vi "GenFPGActrlRef.vi"(4 "DSA excitation":dbl, 6 "Ref Ch.":T2, 7 "Current Time [s]":dbl, 8 "error in (no error)":errorcluster, 9 "Z,ThX,ThY Ref_Cluster":T3 {"Twist_ref [V]" step=0.1; "Bend_ref [V]" step=0.1}, 10 "Reference Offset":T4={"phase"=0.0, "amplitude"=1.0, "frequency"=1.0, "offset"=1.0, "Signal"=enum."Sine"} {"offset" format="%0.2f"; "frequency" format="%0.2f"; "amplitude" format="%0.2f"; "phase" format="%0.2f"}, 11 "FPGA Interface":T1) -> (0 "error out":errorcluster, 2 "Ref Signal":dbl[](array[numeric]), 3 "FPGA VI Reference Out":T1)   [LabVIEW 2017]
doc: "Generate reference signal for the FPGA controller and send params to FPGA"
uses:
  Components/SignalGen/SignalGen.lvlib
  <vilib>/rvi/interface/nirviReadWriteControl/nirviReadWriteControl.xnode
  TypeDefs/FPGA VI Reference.ctl
  FPGA Bitfiles/flexlab_FPGATarget_Tbeamrawv2MainVI_U8ISWGKWIPM.lvbitx
  NiFpgaLv.dll
  <vilib>/Utility/error.llb/Error Cluster From Error Code.vi
  <vilib>/rvi/errors/niLvFpgaAdjustHostInterfaceError.vi
  Components/SignalGen/SignalGenParams_Cluster.ctl
  TypeDefs/BendTwist_Ref_Cluster.ctl
  TypeDefs/RefChEnum.ctl
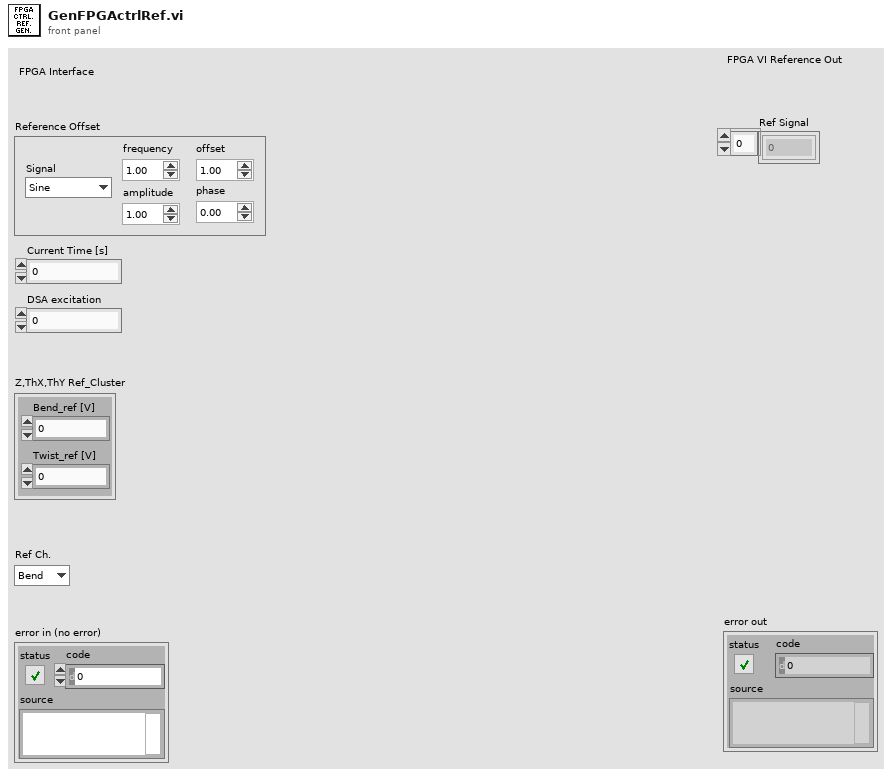
[diagram p1: front panel]
types:
  T1 = typedef "FPGA VI Reference.ctl" = refnum<k20>
  T2 = typedef "RefChEnum.ctl" = enum16{"Bend", "Twist"}
  T3 = typedef "BendTwist_Ref_Cluster.ctl" = cluster{"Bend_ref [V]":dbl, "Twist_ref [V]":dbl}
  T4 = typedef "SignalGen.lvlib/SignalGenParams_Cluster.ctl" = cluster{"phase":dbl, "amplitude":dbl, "frequency":dbl, "offset":dbl, "Signal":enum16{"DC", "Sine", "Square", "Triangle", "Sawtooth", "DSA"}}
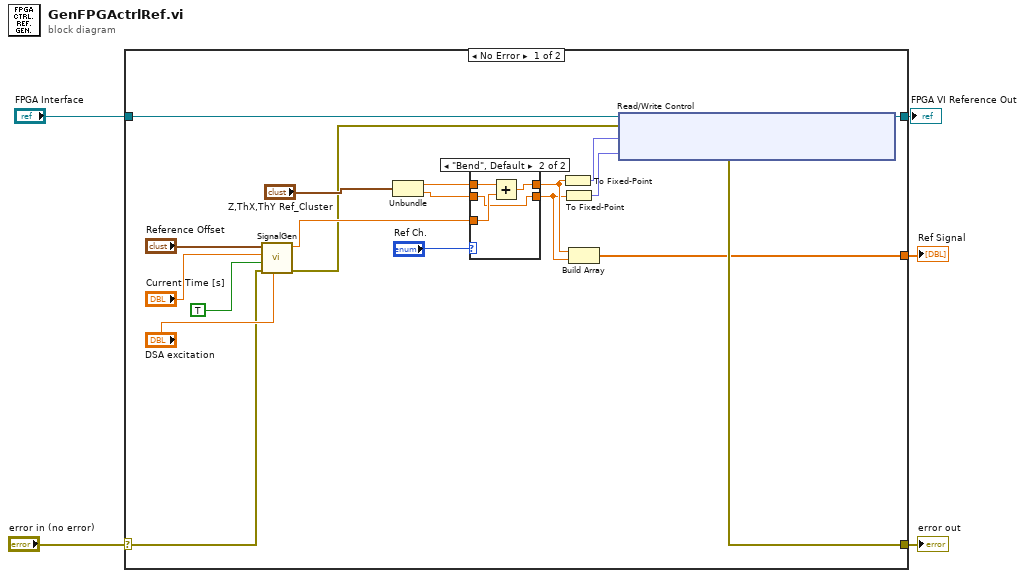
[diagram p0: block diagram]
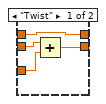
[diagram p2: hidden frame]
diagram:
  n1 = case shown="No Error" "error in (no error)" {
    selector: "error in (no error)" -> [w13 w34]
    tunnel: [w12 w34] -> w4
    tunnel: [w15 w33] -> w3
    tunnel: "FPGA Interface" -> [w16 w33]
    tunnel: [w9 _] -> w2
    frame No Error {
      n2 = call "SignalGen.vi"("DSA excitation"="DSA excitation", "error in (no error)"=w13, "Enable?"=TRUE, "Current Time [s]"="Current Time [s]", "Signal Cluster"="Reference Offset") -> ("error out"=w14:errorcluster, "Signal Out"=w18:dbl)  [unwired: 5 in]
      n3 = Unbundle("Z,ThX,ThY Ref_Cluster") -> ("Bend_ref [V]"=w19:dbl, "Twist_ref [V]"=w8:dbl)
      n4 = case shown="\"Bend\", Default" "Ref Ch." {
        tunnel: w18 -> [w28 w32]
        tunnel: w19 -> [w26 w31]
        tunnel: w8 -> [w27 w29]
        tunnel: [w26 w30] -> w11
        tunnel: [w25 w29] -> w10
        frame "Twist" {
          n5 = Add(x=w27, y=w28) -> (x+y=w25:dbl)
        }
        frame "Bend", Default {
          n6 = Add(x=w31, y=w32) -> (x+y=w30:dbl)
        }
      }
      n7 = To Fixed-Point(number=w11) -> (fixed-point=w7:fxp<+/-,26,4>)  [unwired: 1 in]
      n8 = To Fixed-Point(number=w10) -> (fixed-point=w6:fxp<+/-,26,4>)  [unwired: 1 in]
      n9 = Build Array(w11, w10) -> (w9:dbl[])
      n10 = xnode "Read/Write Control"("FPGA VI Reference In"=w16, "error in"=w14, "Bend reference [V]"=w7, "Twist reference [V]"=w6) -> ("FPGA VI Reference Out"=w15:T1, "error out"=w12:errorcluster)
    }
    frame Error {
    }
  }
  "error out" <- w4
  "FPGA VI Reference Out" <- w3
  "Ref Signal" <- w2
